vi "get_open_closed_pixels.vi"(8 "error in (no error)":errorcluster, 11 "TrajectoryDL090201FrameScan in":refnum<class "TrajectoryDL090201FrameScan.lvclass">) -> (0 "error out":errorcluster, 1 "number of closed pixels":i32, 2 "number of open pixels":i32, 3 "TrajectoryDL090201FrameScan out":refnum<class "TrajectoryDL090201FrameScan.lvclass">, 5 "number of offset pixels":i32)   [LabVIEW 2010, in "TrajectoryDL090201FrameScan.lvclass"]
uses:
  TrajectoryDL090201FrameScan.lvclass
  TrajectoryDL090201FrameScan.lvclass/TrajectoryDL090201FrameScan.ctl
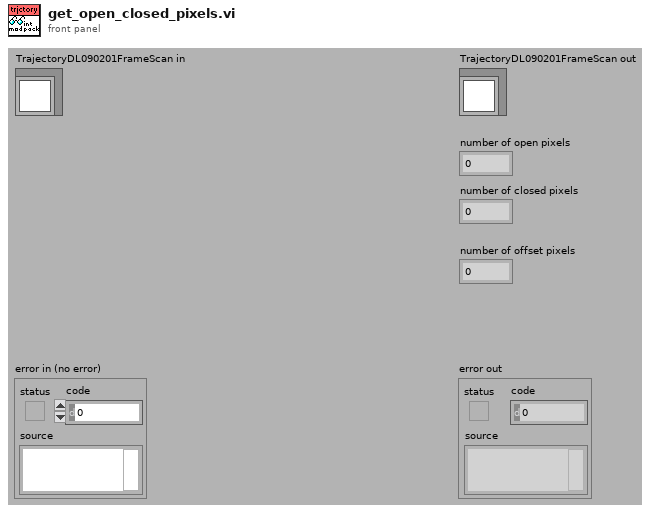
[diagram p1: front panel]
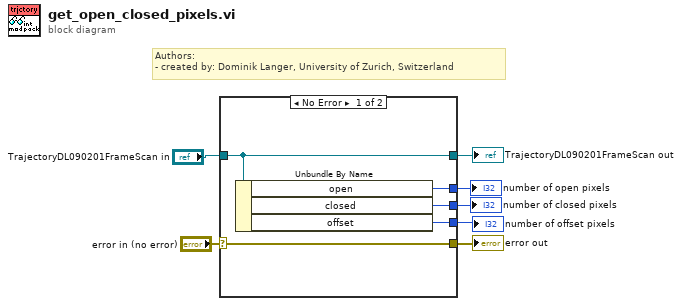
[diagram p0: block diagram]
diagram:
  # "Authors: \n- created by: Dominik Langer, University of Zurich, Switzerland"
  n1 = case shown="No Error" "error in (no error)" {
    selector: "error in (no error)" -> [w12 w14]
    tunnel: [w12 w14] -> w6
    tunnel: [w11 w13] -> w4
    tunnel: "TrajectoryDL090201FrameScan in" -> [w11 w13]
    tunnel: [w10 _] -> w3
    tunnel: [w9 _] -> w2
    tunnel: [w8 _] -> w1
    frame No Error {
      n2 = Unbundle By Name(w11) -> ("open"=w10:i32, "closed"=w9:i32, "offset"=w8:i32)
    }
    frame Error {
    }
  }
  "error out" <- w6
  "TrajectoryDL090201FrameScan out" <- w4
  "number of open pixels" <- w3
  "number of closed pixels" <- w2
  "number of offset pixels" <- w1
